vi "hardware_initialize_hardware.vi"(8 "error in (no error)":errorcluster, 11 "newport_xps in":refnum<class "newport_xps.lvclass">) -> (0 "error out":errorcluster, 3 "newport_xps out":refnum<class "newport_xps.lvclass">)   [LabVIEW 2015, in "newport_xps.lvclass"]
uses:
  newport_xps.lvclass
  newport_xps.lvclass/newport_xps.ctl
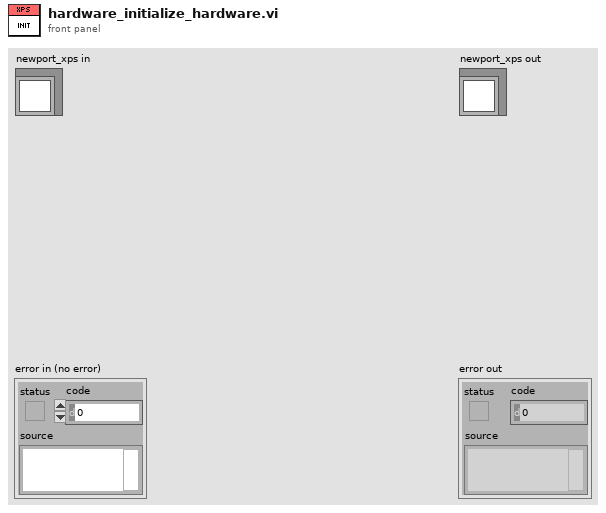
[diagram p1: front panel]
types:
  T1 = cluster{"connection TCP":refnum<k5>, "LogTo File":bool, "Log File refnum":refnum<file>, "no error if error log":bool}
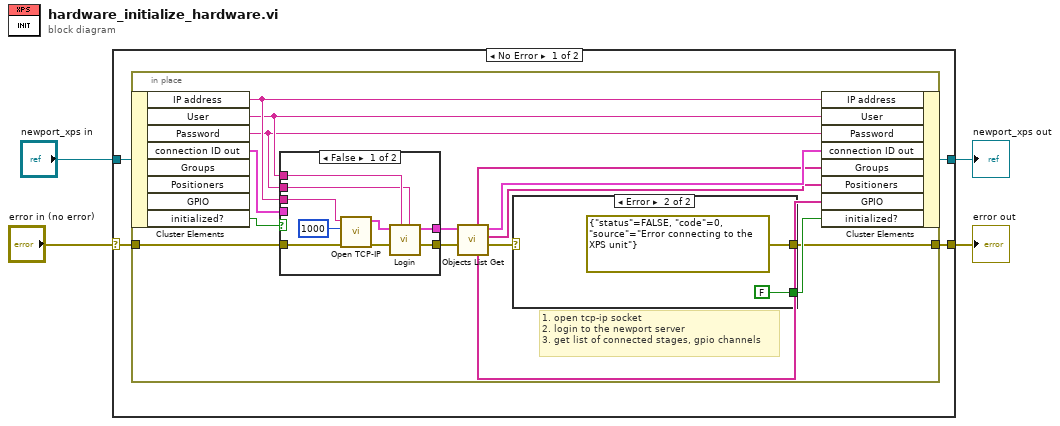
[diagram p0: block diagram]
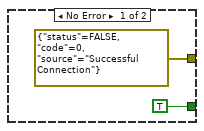
[diagram p3: hidden frame]
diagram:
  n1 = case shown="No Error" "error in (no error)" {
    selector: "error in (no error)" -> [w7 w40]
    tunnel: "newport_xps in" -> [w8 w39]
    tunnel: [w6 w40] -> w2
    tunnel: [w5 w39] -> w1
    frame No Error {
      n2 = in-place {
        in-place-border: w7 -> [w23]
        in-place-border: [w11] -> w6
        # "1. open tcp-ip socket\n2. login to the newport server\n3. get list of connected stages, gpio channels"
        n3 = in-place-cluster #1(w8) -> ("IP address"=w20:string, "User"=w19:string, "Password"=w18:string, "connection ID out"=w9:T1, "initialized?"=w10:bool)  [unwired: 3 out]
        n4 = case shown="False" w10 {
          tunnel: w23 -> [w32 w33]
          tunnel: [w29 w33] -> w22
          tunnel: [w28 w34] -> w21
          tunnel: w20 -> [w27 _]
          tunnel: w19 -> [w26 _]
          tunnel: w18 -> [w25 _]
          tunnel: w9 -> [_ w34]
          frame False {
            n5 = call "Open TCP-IP.vi"("error in (no error)"=w32, "timeout ms (60000)"=1000, "IP address"=w27) -> ("error out"=w30:errorcluster, "Connection ID"=w31:T1)  [unwired: 6 in, 1 out]
            n6 = call "Login.vi"("Password"=w25, "User"=w26, "XPS error in (no error)"=w30, "connection ID in"=w31) -> ("XPS error out"=w29:errorcluster, "connection ID out"=w28:T1)  [unwired: 5 in, 1 out]
          }
          frame True {
          }
        }
        n7 = call "Objects List Get.vi"("XPS error in (no error)"=w22, "connection ID in"=w21) -> ("XPS error out"=w13:errorcluster, "Positioners"=w15:string[], "connection ID out"=w17:T1, "GPIO"=w14:string[], "Groups"=w16:string[])  [unwired: 4 in, 1 out]
        n8 = case shown="Error" w13 {
          tunnel: [TRUE FALSE] -> w12
          tunnel: [errorcluster {"status"=FALSE, "code"=0, "source"="Successful Connection"} ("error IO") errorcluster {"status"=FALSE, "code"=0, "source"="Error connecting to the XPS unit"} ("error IO")] -> w11
          frame No Error {
          }
          frame Error {
          }
        }
        n9 = in-place-cluster #1("IP address"=w20, "User"=w19, "Password"=w18, "connection ID out"=w17, "Groups"=w16, "Positioners"=w15, "GPIO"=w14, "initialized?"=w12) -> (w5:refnum<class "newport_xps.lvclass">)
      }
    }
    frame Error {
    }
  }
  "error out" <- w2
  "newport_xps out" <- w1
